vi "Write PhaseArray.vi"(8 "error in (no error)":errorcluster, 10 "PhaseArray":T1[](array[typedef])=[enum."VA", enum."VB", enum."VC", enum."V+", enum."IA", enum."IB", enum."IC", enum."I+"], 11 "PmuBase in":refnum<class "PmuBase.lvclass">) -> (0 "error out":errorcluster, 3 "PmuBase out":refnum<class "PmuBase.lvclass">)   [LabVIEW 2014, in "SensorPlugins.lvlib" / "PmuBase.lvclass"]
uses:
  PmuBase.lvclass
  Typedef/ePhases.ctl
  PmuBase.lvclass/PmuBase.ctl
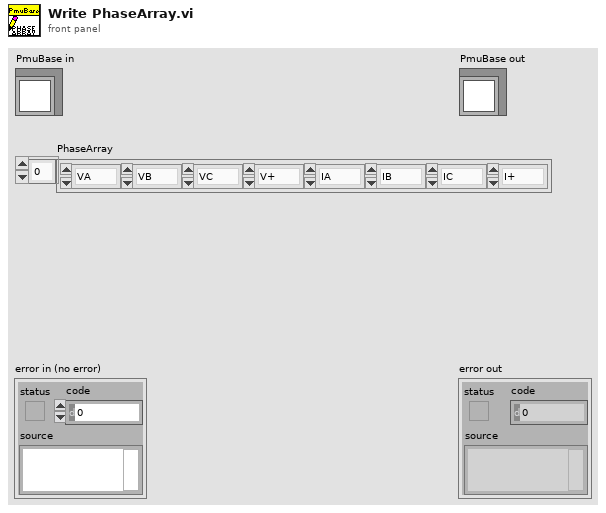
[diagram p1: front panel]
types:
  T1 = typedef "SensorPlugins.lvlib/PmuBase.lvclass/ePhases.ctl" = enum16{"VA", "VB", "VC", "V+", "IA", "IB", "IC", "I+", "none"}
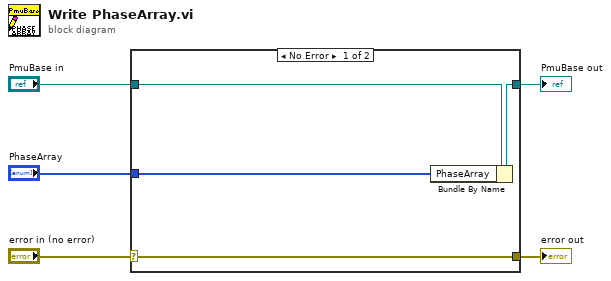
[diagram p0: block diagram]
diagram:
  n1 = case shown="No Error" "error in (no error)" {
    selector: "error in (no error)" -> [w9 w10]
    tunnel: [w9 w10] -> w4
    tunnel: [w7 w11] -> w2
    tunnel: "PmuBase in" -> [w8 w11]
    tunnel: "PhaseArray" -> [w6 _]
    frame No Error {
      n2 = Bundle By Name(cluster=w8, "PhaseArray"=w6) -> (w7:refnum<class "PmuBase.lvclass">)
    }
    frame Error {
    }
  }
  "error out" <- w4
  "PmuBase out" <- w2
